vi "Gen.Network.vi"(8 "error in (no error)":errorcluster) -> (0 "error out":errorcluster)   [LabVIEW 2020]
doc: "Network for GeneralPurposes\n\ninput:\n -- error in -- cluster\n\noutput:\n --error out -- cluster"
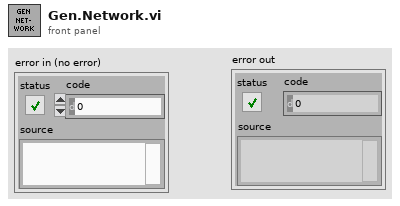
[diagram p1: front panel]
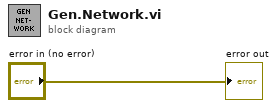
[diagram p0: block diagram]
diagram:
  "error out" <- "error in (no error)"
